vi "Admin (2).vi"() -> ()   [LabVIEW 2020]
panel:
  out "Ban":i32
  out "Tab Control":enum32{"Login", "Admin"}(tab)
  in  "Ingresar":bool
  in  "Contraseña":string
  in  "Usuario":string
  in  "Terminar":bool
  in  "AddContraseña":string
  in  "addUsuario":string
  in  "Agregar":bool
  out "Sesion Iniciada Por:":string
  in  "Volver":bool
  in  "Lista":bool
  out "String":string
  in  "Eliminar":bool
  in  "Ingrese el usuario que desea eliminar":string
  in  "Borrar":bool
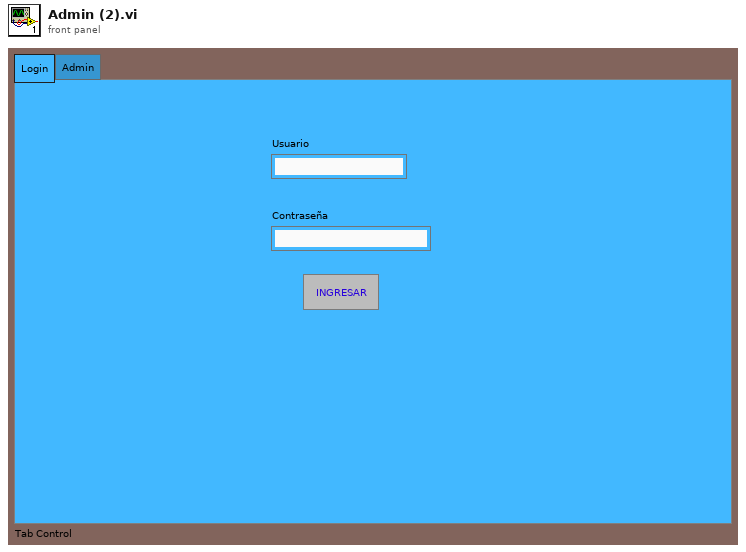
[diagram p1: front panel]
types:
  T1 = enum16{"open", "replace", "create", "open or create", "replace or create", "replace or create with confirmation"}
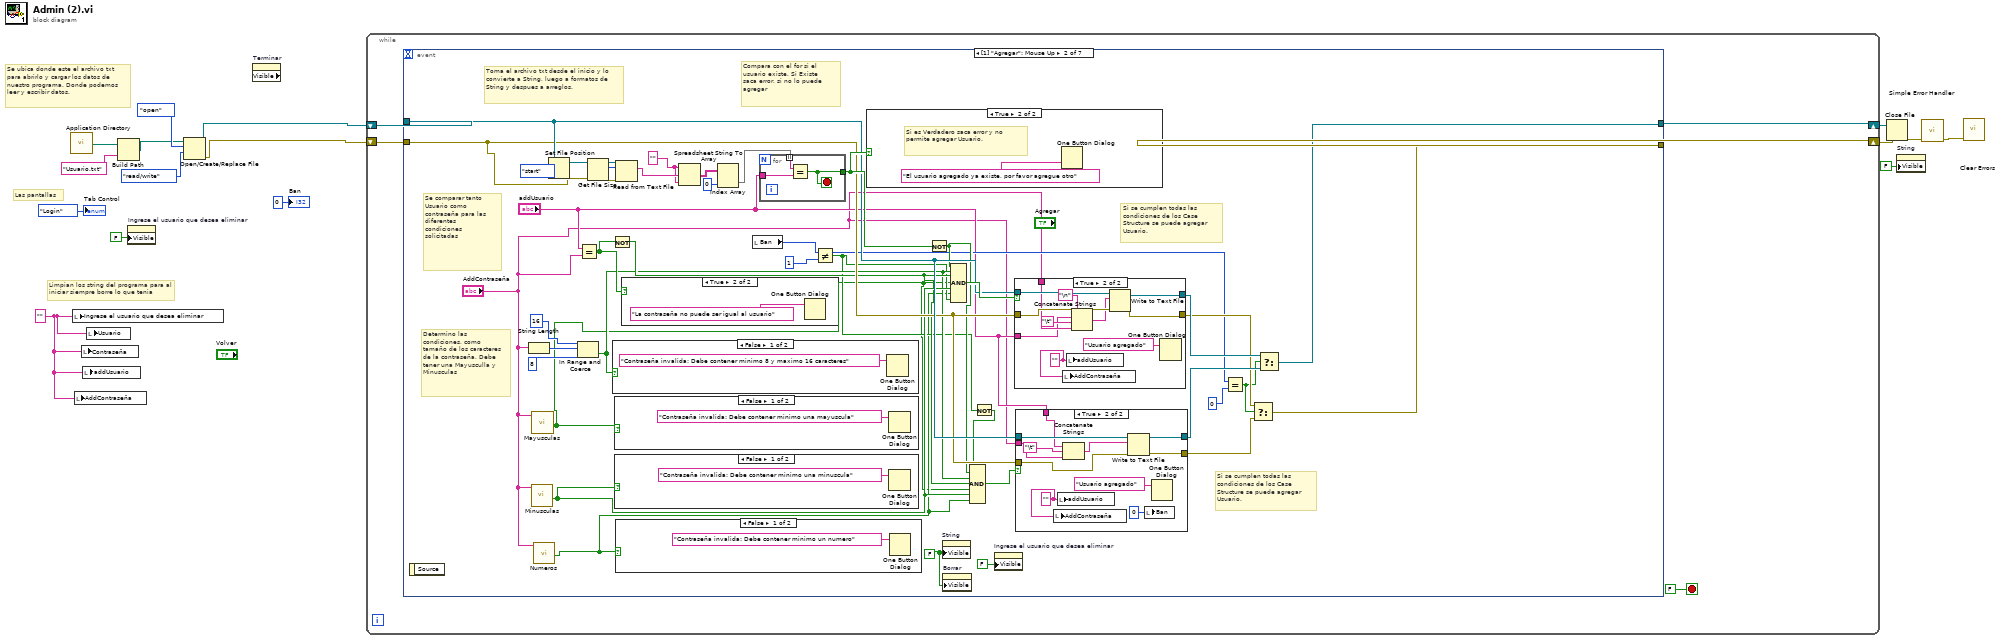
[diagram p0: block diagram]
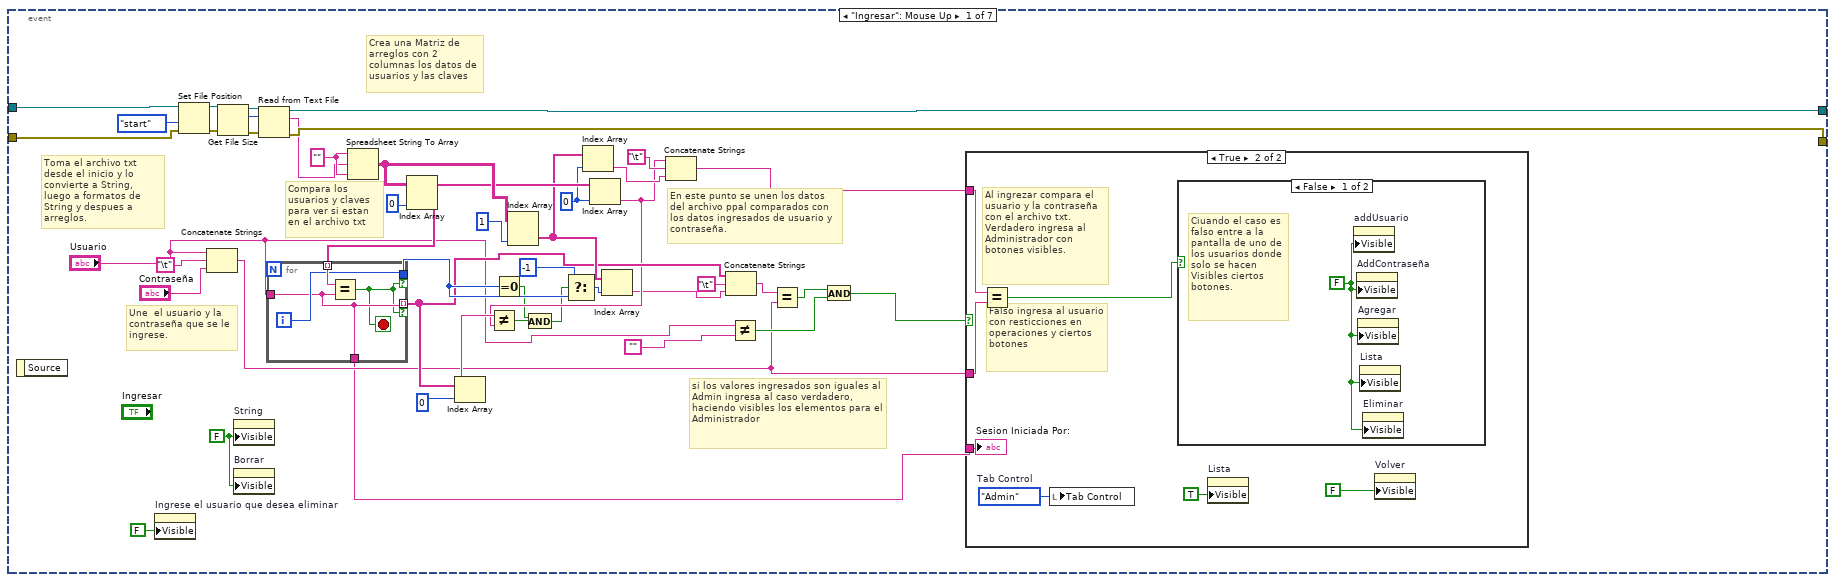
[diagram p2: hidden frame]
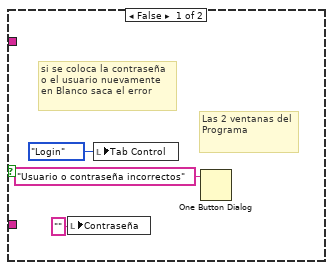
[diagram p3: hidden frame]
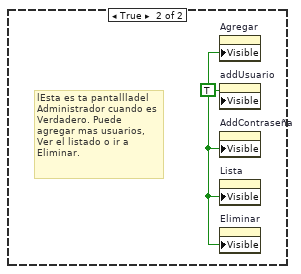
[diagram p4: hidden frame]
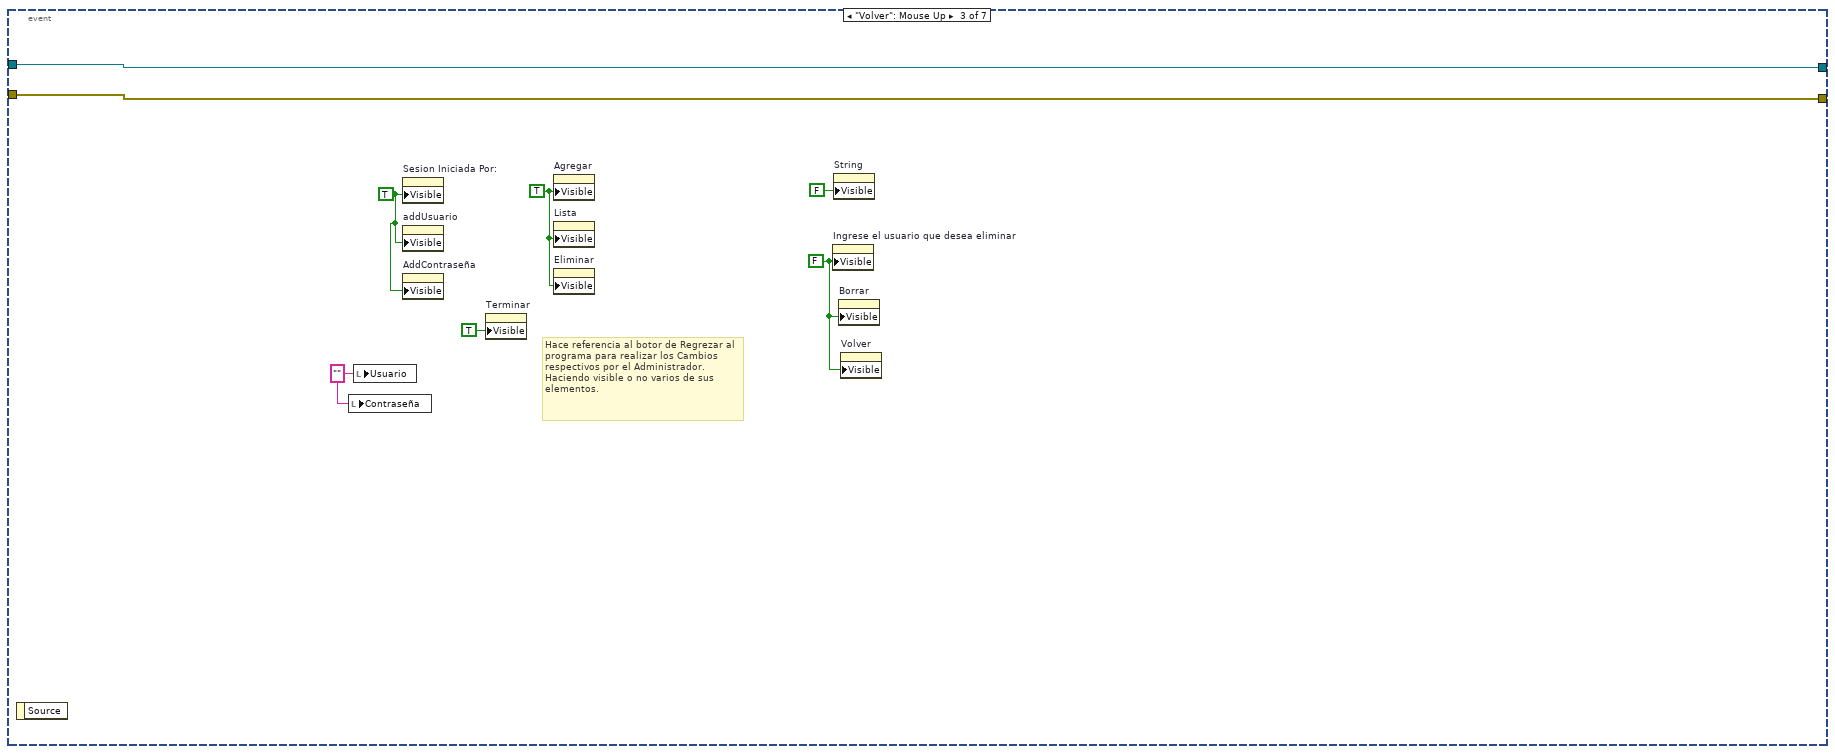
[diagram p13: hidden frame]
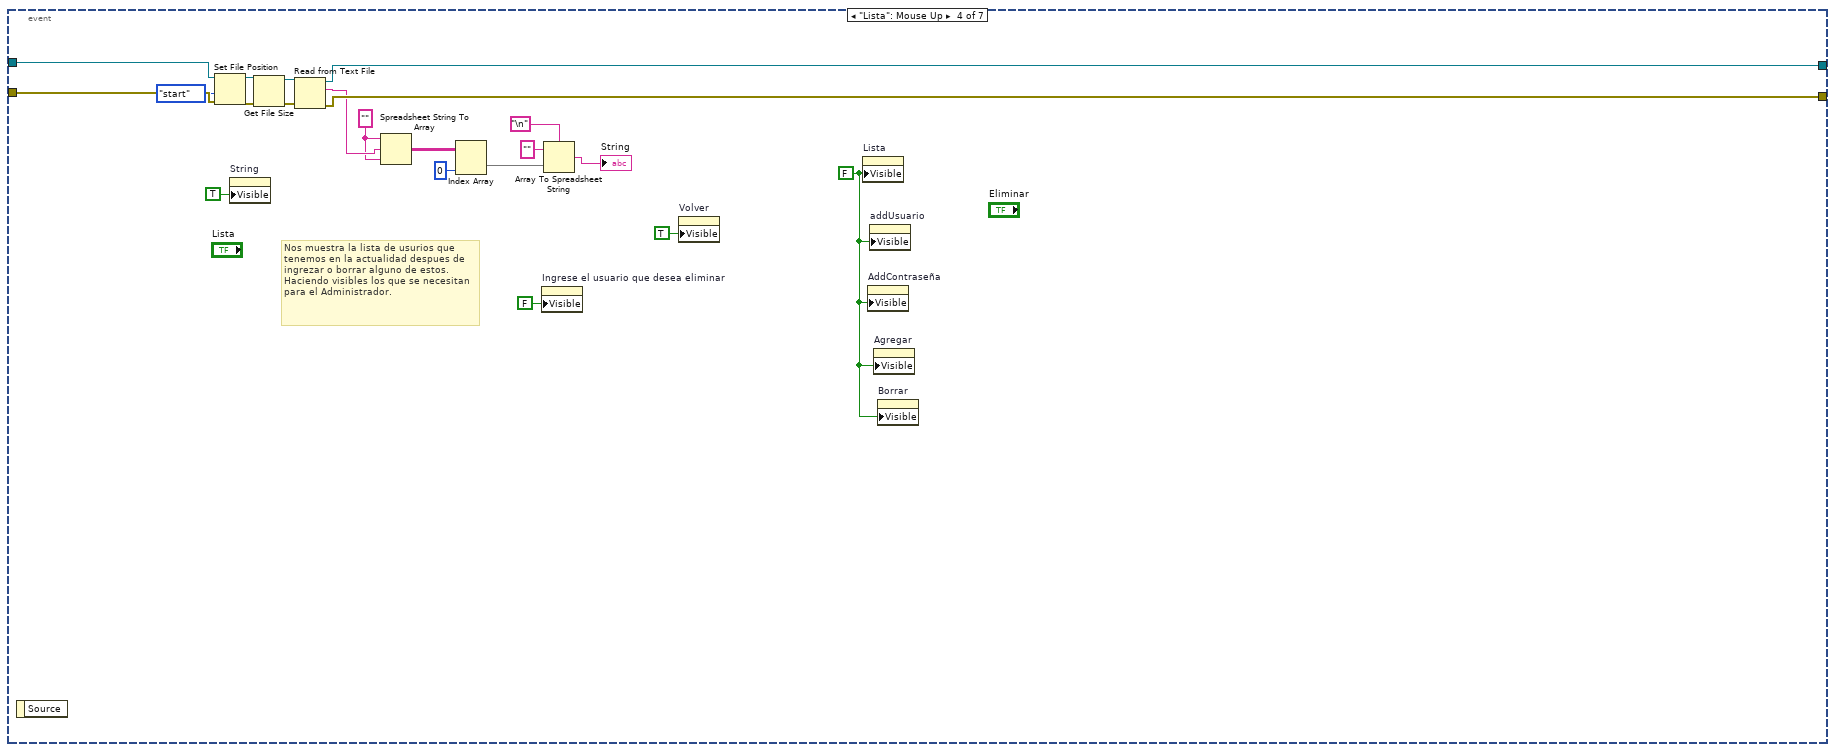
[diagram p14: hidden frame]
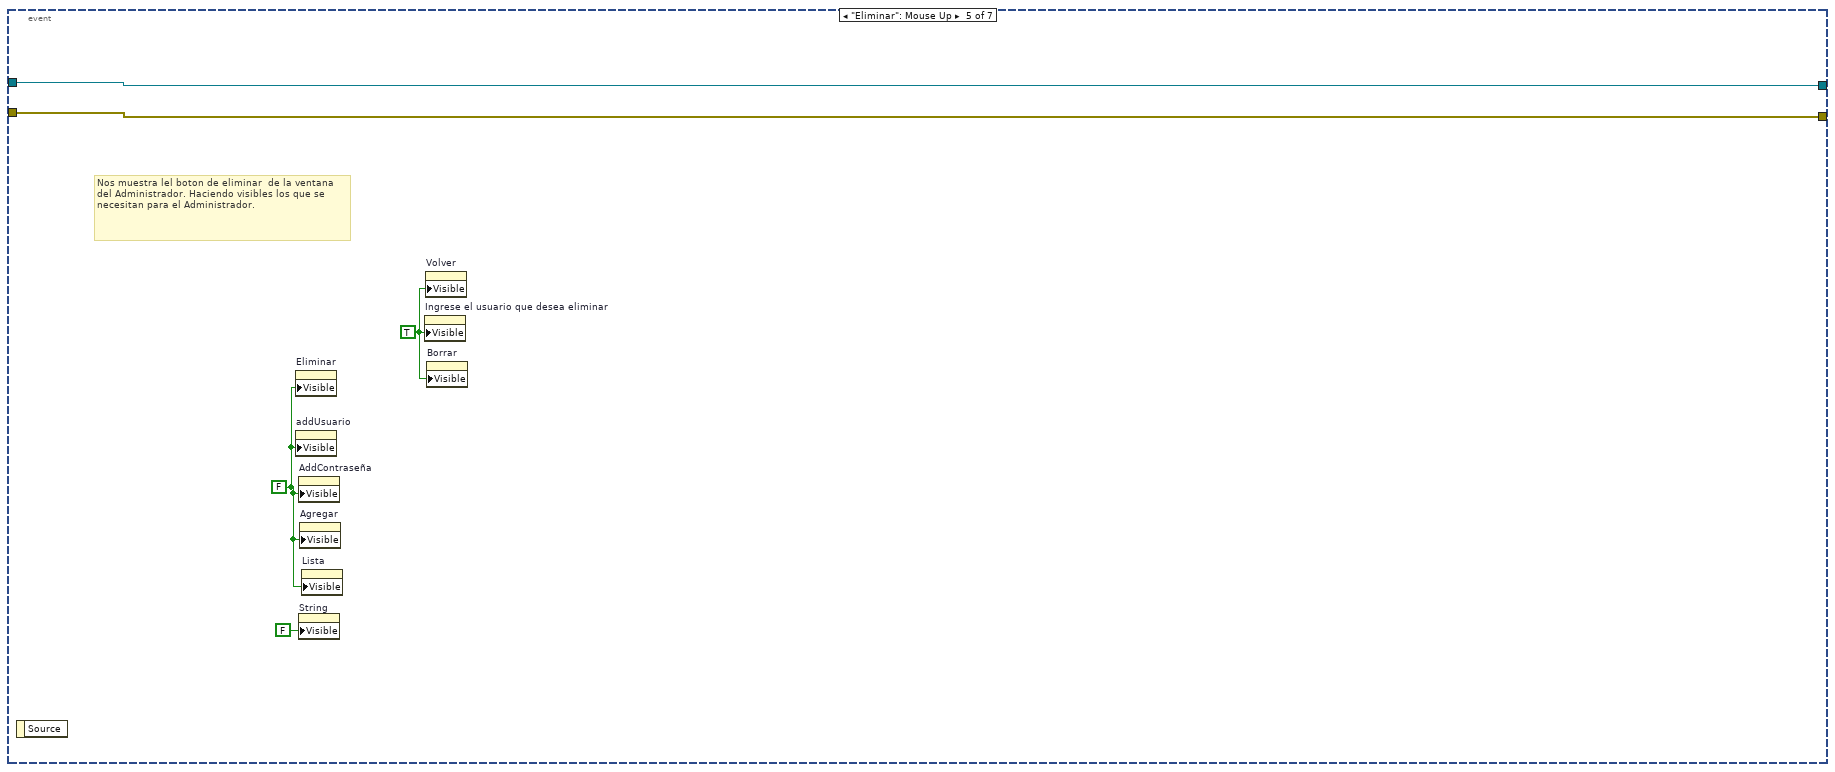
[diagram p15: hidden frame]
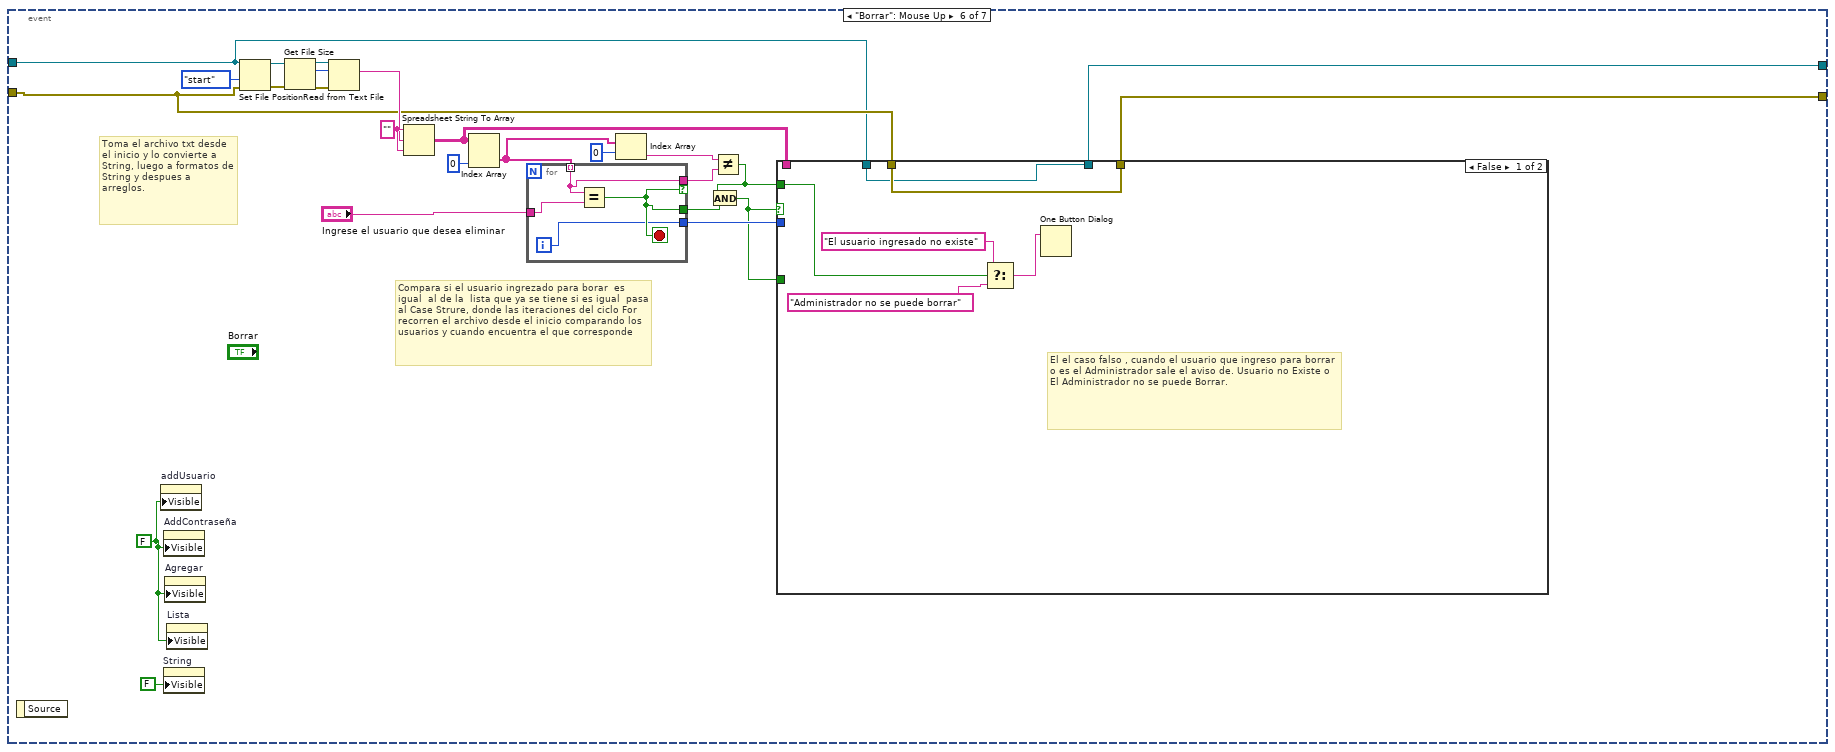
[diagram p16: hidden frame]
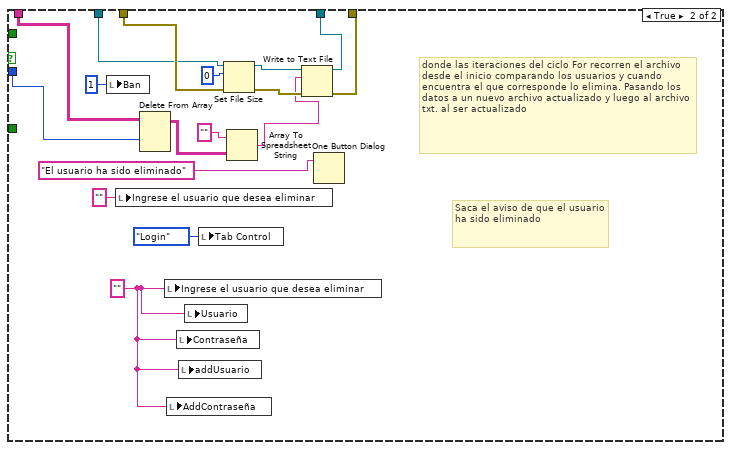
[diagram p17: hidden frame]
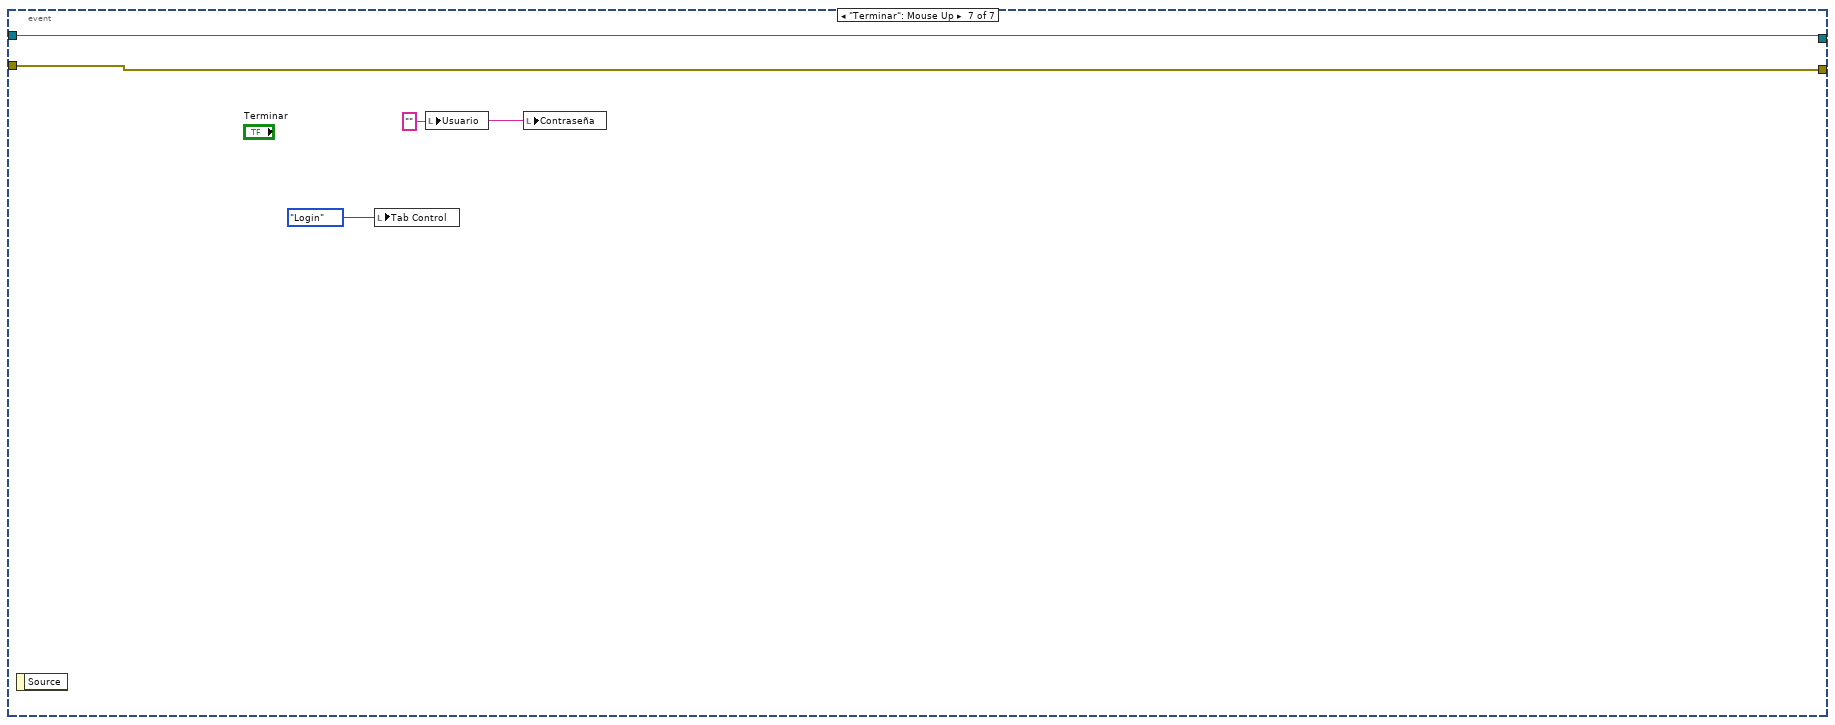
[diagram p18: hidden frame]
diagram:
  w6 = "" ("Usuario")
  # "Las pantallas"
  # "Limpian los string del programa para al iniciar siempre borre lo que tenia"
  # "Se ubica donde este el archivo txt para abrirlo y cargar los datos de nuestro programa. Donde podemos leer y escribir datos."
  n1 = call <vilib>:"Application Directory.vi"() -> ("Application Directory"=w16:path)
  n2 = local write "Ingrese el usuario que desea eliminar"(w6) -> ()
  n3 = local write "AddContraseña"(w6) -> ()
  n4 = local write "Contraseña"(w6) -> ()
  n5 = local write "addUsuario"(w6) -> ()
  n6 = local write "Usuario"(w6) -> ()
  n7 = Build Path(base path=w16, name or relative path="Usuario.txt") -> (appended path=w1:path)
  n8 = property on="Ingrese el usuario que desea eliminar" class="Str"("Visible"=FALSE) -> ()  [unwired: 2 in, 2 out]
  n9 = Open/Create/Replace File(file path (use dialog)=w1, operation (0:open)=T1."open", access (0:read/write)=enum16{"read/write", "read-only", "write-only"}."read/write") -> (refnum out=w4:refnum<file>, error out=w5:errorcluster)  [unwired: 3 in, 1 out]
  n10 = property on="Terminar" class="Bool (strict)" props=["Visible"]() -> ()  [unwired: 2 in, 3 out]
  n11 = while {
    shift-right: [w18] -> w10
    shift-left: w4 -> [w20]
    shift-right: [w17] -> w9
    shift-left: w5 -> [w19]
    stop <- FALSE stop-if-true
    n12 = event shown="[1] \"Agregar\": Mouse Up" {
      selector: _ -> [_ _ _ _ _ _ _]
      dyn-events: _ -> [_ _ _ _ _ _ _]
      timeout: _ -> [_ _ _ _ _ _ _]
      tunnel: w20 -> [w66 w104 w166 w186 w193 w203 w248]
      tunnel: w19 -> [w64 w103 w165 w183 w192 w204 w247]
      tunnel: [w42 w93 w166 w168 w193 w201 w248] -> w18
      tunnel: [w58 w90 w165 w181 w192 w202 w247] -> w17
      event "Ingresar": Mouse Up {
        w43 = FALSE ("Visible")
        w49 = 0 ("index")
        w56 = "" ("format string")
        # "En este punto se unen los datos del archivo ppal comparados con  los datos ingresados de usuario y contraseña."
        # "si los valores ingresados son iguales al  Admin ingresa al caso verdadero, haciendo visibles los elementos para el Administrador"
        # "Compara los usuarios y claves para ver si estan en el archivo txt"
        # "Une  el usuario y la contraseña que se le ingrese."
        # "Crea una Matriz de arreglos con 2 columnas los datos de usuarios y las claves"
        # "Toma el archivo txt desde el inicio y lo convierte a String, luego a formatos de String y despues a arreglos."
        n13 = event-data() -> ()  [unwired: 1 in, 1 out]
        n14 = property on="Ingrese el usuario que desea eliminar" class="Str"("Visible"=FALSE) -> ()  [unwired: 2 in, 2 out]
        n15 = Set File Position(refnum=w66, from (0:start)=enum16{"start", "end", "current"}."start", error in=w64) -> (refnum out=w62:refnum<file>, error out=w63:errorcluster)  [unwired: 1 in]
        n16 = Concatenate Strings "Concatenate Strings"("Usuario", "\t", "Contraseña") -> (w28:string)
        n17 = Get File Size(file=w62, error in=w63) -> (refnum out=w61:refnum<file>, size (in bytes)=w60:i64, 0:w59:errorcluster)
        n18 = property on="String" class="Str"("Visible"=w43) -> ()  [unwired: 2 in, 2 out]
        n19 = property on="Borrar" class="Bool (strict)"("Visible"=w43) -> ()  [unwired: 2 in, 2 out]
        n20 = Read from Text File(file (use dialog)=w61, count=w60, error in=w59) -> (refnum out=w42:refnum<file>, text=w53:string, error out=w58:errorcluster)  [unwired: 1 in, 1 out]
        n21 = Spreadsheet String To Array(format string=w56, spreadsheet string=w53, array type (2D Dbl)=w56) -> (array=w51:string[][])  [unwired: 1 in]
        n22 = Index Array "Index Array"(array=w51, index (col)=0 ("disabled index (col)")) -> (element=w50:string[])  [unwired: 1 in]
        n23 = for {
          tunnel: w50 -> [w70] mode=indexing
          tunnel: "Usuario" -> [w68]
          tunnel: [w68] -> w38 mode=indexing if=w67
          tunnel: [w69] -> w40 if=w67
          tunnel: [w68] -> w22
          i -> [w69]
          stop <- w67 stop-if-true
          n24 = Equal?(x=w70, y=w68) -> (x = y?=w67:bool)
        }
        n25 = Index Array "Index Array"(array=w38, index=0) -> (element=w36:string)
        n26 = Equal To 0?(x=w40) -> (x = 0?=w33:bool)
        n27 = Index Array "Index Array"(array=w51, index (col)=1 ("disabled index (col)")) -> (element=w45:string[])  [unwired: 1 in]
        n28 = Index Array "Index Array"(array=w45, index=w49) -> (element=w48:string)
        n29 = Index Array(array=w50, index=w49) -> (element=w35:string)
        n30 = Not Equal?(x=w36, y=w35) -> (x != y?=w34:bool)
        n31 = And(x=w33, y=w34) -> (x .and. y?=w32:bool)
        n32 = Select(t=-1, s=w32, f=w40) -> (s? t:f=w39:i32)
        n33 = Index Array(array=w45, index=w39) -> (element=w25:string)
        n34 = Concatenate Strings(w35, "\t", w48) -> (w46:string)
        n35 = Concatenate Strings "Concatenate Strings"(w38, "\t", w25) -> (w29:string)
        n36 = Not Equal?(x="Usuario", y="") -> (x != y?=w31:bool)
        n37 = Equal?(x=w29, y=w28) -> (x = y?=w26:bool)
        n38 = And(x=w26, y=w31) -> (x .and. y?=w30:bool)
        n39 = case shown="True" w30 {
          tunnel: w28 -> [_ w80]
          tunnel: w46 -> [_ w79]
          tunnel: w22 -> [_ w78]
          frame False {
            # "Las 2 ventanas del   Programa"
            # "si se coloca la contraseña o el usuario nuevamente en Blanco saca el error"
            n40 = local write "Contraseña"("" ("Usuario")) -> ()
            n41 = local write "Tab Control"(enum32{"Login", "Admin"}."Login" ("Tab Control")) -> ()
            n42 = One Button Dialog(message="Usuario o contraseña incorrectos") -> ()  [unwired: 1 in, 1 out]
          }
          frame True {
            w75 = enum32{"Login", "Admin"}."Admin"  # Tab Control
            # "Falso ingresa al usuario con resticciones en operaciones y ciertos botones"
            # "Al ingrezar compara el usuario y la contraseña con el archivo txt.  Verdadero ingresa al Administrador con botones visibles."
            n43 = Equal?(x=w79, y=w80) -> (x = y?=w76:bool)
            n44 = local write "Tab Control"(w75) -> ()
            n45 = case shown="False" w76 {
              frame False {
                w81 = FALSE ("Visible")
                # "Ciuando el caso es falso entre a la pantalla de uno de los usuarios donde  solo se hacen Visibles ciertos botones."
                n46 = property on="addUsuario" class="Str"("Visible"=w81) -> ()  [unwired: 2 in, 2 out]
                n47 = property on="AddContraseña" class="Str"("Visible"=w81) -> ()  [unwired: 2 in, 2 out]
                n48 = property on="Agregar" class="Bool (strict)"("Visible"=w81) -> ()  [unwired: 2 in, 2 out]
                n49 = property on="Lista" class="Bool (strict)"("Visible"=w81) -> ()  [unwired: 2 in, 2 out]
                n50 = property on="Eliminar" class="Bool (strict)"("Visible"=w81) -> ()  [unwired: 2 in, 2 out]
              }
              frame True {
                w82 = TRUE ("Visible")
                # "lEsta es ta pantallladel Administrador cuando es Verdadero. Puede agregar mas usuarios, Ver el listado o ir a Eliminar."
                n51 = property on="Agregar" class="Bool (strict)"("Visible"=w82) -> ()  [unwired: 2 in, 2 out]
                n52 = property on="addUsuario" class="Str"("Visible"=w82) -> ()  [unwired: 2 in, 2 out]
                n53 = property on="AddContraseña" class="Str"("Visible"=w82) -> ()  [unwired: 2 in, 2 out]
                n54 = property on="Lista" class="Bool (strict)"("Visible"=w82) -> ()  [unwired: 2 in, 2 out]
                n55 = property on="Eliminar" class="Bool (strict)"("Visible"=w82) -> ()  [unwired: 2 in, 2 out]
              }
            }
            n56 = property on="Lista" class="Bool (strict)"("Visible"=TRUE) -> ()  [unwired: 2 in, 2 out]
            n57 = property on="Volver" class="Bool (strict)"("Visible"=FALSE) -> ()  [unwired: 2 in, 2 out]
            "Sesion Iniciada Por:" <- w78
          }
        }
      }
      event "Agregar": Mouse Up {
        w106 = FALSE ("Visible")
        w112 = "" ("format string")
        # "Si se cumplen todas las condiciones de los Case Structure se puede agregar Usuario."
        # "Si se cumplen todas las condiciones de los Case Structure se puede agregar Usuario."
        # "Determino las condiciones, como tamaño de los caracteres de la contraseña, Debe tener una Mayusculla y Minusculas"
        # "Se comparar tanto Usuario como contraseña para las diferentes condiciones solicitadas"
        # "Compara con el for si el usuario existe. Si Existe saca error, si no lo puede agregar"
        # "Toma el archivo txt desde el inicio y lo convierte a String, luego a formatos de String y despues a arreglos."
        n58 = event-data() -> ()  [unwired: 1 in, 1 out]
        n59 = String Length(string="AddContraseña") -> (length=w122:i32)
        n60 = call "Minusculas.vi"("Palabra"="AddContraseña") -> ("Boolean"=w102:bool)  [unwired: 8 in, 2 out]
        n61 = call "Mayusculas.vi"("Palabra"="AddContraseña") -> ("Boolean"=w83:bool)  [unwired: 8 in, 2 out]
        n62 = call "Numeros.vi"("Palabra"="AddContraseña") -> ("Boolean"=w84:bool)  [unwired: 8 in, 2 out]
        n63 = Set File Position(refnum=w104, from (0:start)=enum16{"start", "end", "current"}."start", error in=w103) -> (refnum out=w115:refnum<file>, error out=w118:errorcluster)  [unwired: 1 in]
        n64 = In Range and Coerce(upper limit=16, x=w122, lower limit=8) -> (In Range?=w100:bool)  [unwired: 1 out]
        n65 = Equal?(x="addUsuario", y="AddContraseña") -> (x = y?=w121:bool)
        n66 = Get File Size(file=w115, error in=w118) -> (refnum out=w116:refnum<file>, size (in bytes)=w119:i64, 0:w117:errorcluster)
        n67 = Not(x=w121) -> (.not. x?=w101:bool)
        n68 = case shown="False" w100 {
          frame False {
            n69 = One Button Dialog(message="Contraseña invalida: Debe contener minimo 8 y maximo 16 caracteres") -> ()  [unwired: 1 in, 1 out]
          }
          frame True {
          }
        }
        n70 = case shown="False" w83 {
          frame False {
            n71 = One Button Dialog(message="Contraseña invalida: Debe contener minimo una mayuscula") -> ()  [unwired: 1 in, 1 out]
          }
          frame True {
          }
        }
        n72 = case shown="False" w102 {
          frame False {
            n73 = One Button Dialog(message="Contraseña invalida: Debe contener minimo una minuscula") -> ()  [unwired: 1 in, 1 out]
          }
          frame True {
          }
        }
        n74 = Read from Text File(file (use dialog)=w116, count=w119, error in=w117) -> (text=w113:string)  [unwired: 1 in, 3 out]
        n75 = case shown="False" w84 {
          frame False {
            n76 = One Button Dialog(message="Contraseña invalida: Debe contener minimo un numero") -> ()  [unwired: 1 in, 1 out]
          }
          frame True {
          }
        }
        n77 = case shown="True" w121 {
          frame False {
            # "Si no son iguales se pueden agregar al  Programa"
          }
          frame True {
            n78 = One Button Dialog(message="La contraseña no puede ser igual al usuario") -> ()  [unwired: 1 in, 1 out]
          }
        }
        n79 = Spreadsheet String To Array(format string=w112, spreadsheet string=w113, array type (2D Dbl)=w112) -> (array=w111:string[][])  [unwired: 1 in]
        n80 = Index Array(array=w111, index (col)=0 ("disabled index (col)")) -> (element=w109:string[])  [unwired: 1 in]
        n81 = local read "Ban"() -> (w87:i32)
        n82 = for {
          tunnel: "addUsuario" -> [w141]
          tunnel: w109 -> [w140] mode=indexing
          tunnel: [w139] -> w108
          stop <- w139 stop-if-true
          n83 = Equal?(x=w140, y=w141) -> (x = y?=w139:bool)
        }
        n84 = Not Equal?(x=w87, y=1) -> (x != y?=w98:bool)
        n85 = case shown="True" w108 {
          frame False {
            # "Si es Falso lo Puede Agregar ur¿suario en la base de Datos"
          }
          frame True {
            # "Si es Verdadero saca error y no permite agregar Usuario."
            n86 = One Button Dialog(message="El usuario agregado ya existe, por favor agregue otro") -> ()  [unwired: 1 in, 1 out]
          }
        }
        n87 = Not(x=w108) -> (.not. x?=w99:bool)
        n88 = property on="String" class="Str"("Visible"=w106) -> ()  [unwired: 2 in, 2 out]
        n89 = property on="Borrar" class="Bool (strict)"("Visible"=w106) -> ()  [unwired: 2 in, 2 out]
        n90 = Compound Arithmetic op=AND(w99, w100, w101, w83, w102, w84, w98) -> (w120:bool)
        n91 = Not(x=w98) -> (.not. x?=w97:bool)
        n92 = Compound Arithmetic op=AND(w97, w99, w100, w101, w83, w102, w84) -> (w96:bool)
        n93 = property on="Ingrese el usuario que desea eliminar" class="Str"("Visible"=FALSE) -> ()  [unwired: 2 in, 2 out]
        n94 = case shown="True" w120 {
          tunnel: w104 -> [w146 w157]
          tunnel: w103 -> [w145 w156]
          tunnel: [w146 w155] -> w95
          tunnel: [w145 w154] -> w92
          tunnel: "addUsuario" -> [_ w147]
          tunnel: "AddContraseña" -> [_ w153]
          frame False {
          }
          frame True {
            w148 = "" ("addUsuario")
            n95 = local write "AddContraseña"(w148) -> ()
            n96 = local write "addUsuario"(w148) -> ()
            n97 = Concatenate Strings("\n", w147, "\t", w153) -> (w152:string)
            n98 = Write to Text File(file (use dialog)=w157, text=w152, error in=w156) -> (refnum out=w155:refnum<file>, error out=w154:errorcluster)  [unwired: 1 in, 1 out]
            n99 = One Button Dialog(message="Usuario agregado") -> ()  [unwired: 1 in, 1 out]
          }
        }
        n100 = case shown="True" w96 {
          tunnel: w104 -> [w126 w133]
          tunnel: w103 -> [w125 w132]
          tunnel: [w126 w131] -> w94
          tunnel: [w125 w130] -> w91
          tunnel: "addUsuario" -> [_ w128]
          tunnel: "AddContraseña" -> [_ w127]
          frame False {
          }
          frame True {
            w137 = "" ("addUsuario")
            n101 = local write "AddContraseña"(w137) -> ()
            n102 = local write "addUsuario"(w137) -> ()
            n103 = Concatenate Strings(w128, "\t", w127) -> (w135:string)
            n104 = Write to Text File(file (use dialog)=w133, text=w135, error in=w132) -> (refnum out=w131:refnum<file>, error out=w130:errorcluster)  [unwired: 1 in, 1 out]
            n105 = local write "Ban"(0 ("Ban")) -> ()
            n106 = One Button Dialog(message="Usuario agregado") -> ()  [unwired: 1 in, 1 out]
          }
        }
        n107 = Equal?(x=w87, y=0) -> (x = y?=w88:bool)
        n108 = Select(t=w92, s=w88, f=w91) -> (s? t:f=w90:errorcluster)
        n109 = Select(t=w95, s=w88, f=w94) -> (s? t:f=w93:refnum<file>)
      }
      event "Volver": Mouse Up {
        w162 = TRUE ("Visible")
        w163 = TRUE ("Visible")
        w160 = FALSE ("Visible")
        w167 = "" ("Usuario")
        # "Hace referencia al botor de Regrezar al programa para realizar los Cambios respectivos por el Administrador.  Haciendo visible o no varios de sus elementos."
        n110 = event-data() -> ()  [unwired: 1 in, 1 out]
        n111 = local write "Contraseña"(w167) -> ()
        n112 = local write "Usuario"(w167) -> ()
        n113 = property on="Sesion Iniciada Por:" class="Str"("Visible"=w163) -> ()  [unwired: 2 in, 2 out]
        n114 = property on="addUsuario" class="Str"("Visible"=w163) -> ()  [unwired: 2 in, 2 out]
        n115 = property on="AddContraseña" class="Str"("Visible"=w163) -> ()  [unwired: 2 in, 2 out]
        n116 = property on="Terminar" class="Bool (strict)"("Visible"=TRUE) -> ()  [unwired: 2 in, 2 out]
        n117 = property on="Agregar" class="Bool (strict)"("Visible"=w162) -> ()  [unwired: 2 in, 2 out]
        n118 = property on="Lista" class="Bool (strict)"("Visible"=w162) -> ()  [unwired: 2 in, 2 out]
        n119 = property on="Eliminar" class="Bool (strict)"("Visible"=w162) -> ()  [unwired: 2 in, 2 out]
        n120 = property on="Ingrese el usuario que desea eliminar" class="Str"("Visible"=w160) -> ()  [unwired: 2 in, 2 out]
        n121 = property on="String" class="Str"("Visible"=FALSE) -> ()  [unwired: 2 in, 2 out]
        n122 = property on="Borrar" class="Bool (strict)"("Visible"=w160) -> ()  [unwired: 2 in, 2 out]
        n123 = property on="Volver" class="Bool (strict)"("Visible"=w160) -> ()  [unwired: 2 in, 2 out]
      }
      event "Lista": Mouse Up {
        w170 = FALSE ("Visible")
        w179 = "" ("format string")
        # "Nos muestra la lista de usurios que tenemos en la actualidad despues de ingrezar o borrar alguno de estos. Haciendo visibles los que se necesitan para el Administrador."
        n124 = event-data() -> ()  [unwired: 1 in, 1 out]
        n125 = Set File Position(refnum=w186, from (0:start)=enum16{"start", "end", "current"}."start", error in=w183) -> (refnum out=w188:refnum<file>, error out=w184:errorcluster)  [unwired: 1 in]
        n126 = property on="String" class="Str"("Visible"=TRUE) -> ()  [unwired: 2 in, 2 out]
        n127 = Get File Size(file=w188, error in=w184) -> (refnum out=w187:refnum<file>, 0:w185:errorcluster)  [unwired: 1 out]
        n128 = Read from Text File(file (use dialog)=w187, error in=w185) -> (refnum out=w168:refnum<file>, text=w180:string, error out=w181:errorcluster)  [unwired: 2 in, 1 out]
        n129 = Spreadsheet String To Array(format string=w179, spreadsheet string=w180, array type (2D Dbl)=w179) -> (array=w178:string[][])  [unwired: 1 in]
        n130 = Index Array(array=w178, index (col)=0 ("disabled index (col)")) -> (element=w175:string[])  [unwired: 1 in]
        n131 = property on="Ingrese el usuario que desea eliminar" class="Str"("Visible"=FALSE) -> ()  [unwired: 2 in, 2 out]
        n132 = Array To Spreadsheet String(delimiter (Tab)="\n", array=w175, 3:"" ("format string")) -> (spreadsheet string=→"String":string)
        n133 = property on="Volver" class="Bool (strict)"("Visible"=TRUE) -> ()  [unwired: 2 in, 2 out]
        n134 = property on="Lista" class="Bool (strict)"("Visible"=w170) -> ()  [unwired: 2 in, 2 out]
        n135 = property on="AddContraseña" class="Str"("Visible"=w170) -> ()  [unwired: 2 in, 2 out]
        n136 = property on="addUsuario" class="Str"("Visible"=w170) -> ()  [unwired: 2 in, 2 out]
        n137 = property on="Agregar" class="Bool (strict)"("Visible"=w170) -> ()  [unwired: 2 in, 2 out]
        n138 = property on="Borrar" class="Bool (strict)"("Visible"=w170) -> ()  [unwired: 2 in, 2 out]
      }
      event "Eliminar": Mouse Up {
        w190 = FALSE ("Visible")
        w189 = TRUE ("Visible")
        # "Nos muestra lel boton de eliminar  de la ventana del Administrador. Haciendo visibles los que se necesitan para el Administrador."
        n139 = event-data() -> ()  [unwired: 1 in, 1 out]
        n140 = property on="Eliminar" class="Bool (strict)"("Visible"=w190) -> ()  [unwired: 2 in, 2 out]
        n141 = property on="addUsuario" class="Str"("Visible"=w190) -> ()  [unwired: 2 in, 2 out]
        n142 = property on="AddContraseña" class="Str"("Visible"=w190) -> ()  [unwired: 2 in, 2 out]
        n143 = property on="String" class="Str"("Visible"=FALSE) -> ()  [unwired: 2 in, 2 out]
        n144 = property on="Agregar" class="Bool (strict)"("Visible"=w190) -> ()  [unwired: 2 in, 2 out]
        n145 = property on="Lista" class="Bool (strict)"("Visible"=w190) -> ()  [unwired: 2 in, 2 out]
        n146 = property on="Ingrese el usuario que desea eliminar" class="Str"("Visible"=w189) -> ()  [unwired: 2 in, 2 out]
        n147 = property on="Volver" class="Bool (strict)"("Visible"=w189) -> ()  [unwired: 2 in, 2 out]
        n148 = property on="Borrar" class="Bool (strict)"("Visible"=w189) -> ()  [unwired: 2 in, 2 out]
      }
      event "Borrar": Mouse Up {
        w210 = "" ("format string")
        w218 = FALSE ("Visible")
        # "Compara si el usuario ingrezado para borar  es igual  al de la  lista que ya se tiene si es igual  pasa al Case Strure, donde las iteraciones del ciclo For recorren el archivo desde el inicio comparando los usuarios y cuando encuentra el que corresponde"
        # "Toma el archivo txt desde el inicio y lo convierte a String, luego a formatos de String y despues a arreglos."
        n149 = event-data() -> ()  [unwired: 1 in, 1 out]
        n150 = property on="addUsuario" class="Str"("Visible"=w218) -> ()  [unwired: 2 in, 2 out]
        n151 = property on="AddContraseña" class="Str"("Visible"=w218) -> ()  [unwired: 2 in, 2 out]
        n152 = property on="String" class="Str"("Visible"=FALSE) -> ()  [unwired: 2 in, 2 out]
        n153 = property on="Agregar" class="Bool (strict)"("Visible"=w218) -> ()  [unwired: 2 in, 2 out]
        n154 = property on="Lista" class="Bool (strict)"("Visible"=w218) -> ()  [unwired: 2 in, 2 out]
        n155 = Set File Position(refnum=w203, from (0:start)=enum16{"start", "end", "current"}."start", error in=w204) -> (refnum out=w215:refnum<file>, error out=w214:errorcluster)  [unwired: 1 in]
        n156 = Get File Size(file=w215, error in=w214) -> (refnum out=w213:refnum<file>, size (in bytes)=w211:i64, 0:w212:errorcluster)
        n157 = Read from Text File(file (use dialog)=w213, count=w211, error in=w212) -> (text=w209:string)  [unwired: 1 in, 3 out]
        n158 = Spreadsheet String To Array(format string=w210, spreadsheet string=w209, array type (2D Dbl)=w210) -> (array=w206:string[][])  [unwired: 1 in]
        n159 = Index Array(array=w206, index (col)=0 ("disabled index (col)")) -> (element=w196:string[])  [unwired: 1 in]
        n160 = for {
          tunnel: w196 -> [w244] mode=indexing
          tunnel: "Ingrese el usuario que desea eliminar" -> [w245]
          tunnel: [w243] -> w198
          tunnel: [w244] -> w195 if=w243
          tunnel: [w242] -> w205
          i -> [w242]
          stop <- w243 stop-if-true
          n161 = Equal?(x=w244, y=w245) -> (x = y?=w243:bool)
        }
        n162 = Index Array(array=w196, index=0) -> (element=w199:string)
        n163 = Not Equal?(x=w199, y=w195) -> (x != y?=w194:bool)
        n164 = And(x=w194, y=w198) -> (x .and. y?=w197:bool)
        n165 = case shown="False" w197 {
          tunnel: w206 -> [_ w241]
          tunnel: w205 -> [_ w240]
          tunnel: w204 -> [w224 w237]
          tunnel: w203 -> [w223 w236]
          tunnel: [w224 w239] -> w202
          tunnel: [w223 w238] -> w201
          tunnel: w197 -> [_ _]
          tunnel: w194 -> [w221 _]
          frame False {
            # "El el caso falso , cuando el usuario que ingreso para borrar o es el Administrador sale el aviso de. Usuario no Existe o El Administrador no se puede Borrar."
            n166 = Select(t="El usuario ingresado no existe" ("message"), s=w221, f="Administrador no se puede borrar" ("message")) -> (s? t:f=w219:string)
            n167 = One Button Dialog(message=w219) -> ()  [unwired: 1 in, 1 out]
          }
          frame True {
            w225 = "" ("Usuario")
            # "Saca el aviso de que el usuario ha sido eliminado"
            # "donde las iteraciones del ciclo For recorren el archivo desde el inicio comparando los usuarios y cuando encuentra el que corresponde lo elimina. Pasando los datos a un nuevo archivo actualizado y luego al archivo txt. al ser actualizado"
            n168 = local write "Ban"(1 ("Ban")) -> ()
            n169 = local write "Ingrese el usuario que desea eliminar"("" ("Ingrese el usuario que desea eliminar")) -> ()
            n170 = Delete From Array "Delete From Array"(array=w241, index (row)=w240) -> (array with subset deleted=w235:string[][])  [unwired: 2 in, 1 out]
            n171 = local write "Ingrese el usuario que desea eliminar"(w225) -> ()
            n172 = local write "AddContraseña"(w225) -> ()
            n173 = local write "Contraseña"(w225) -> ()
            n174 = local write "addUsuario"(w225) -> ()
            n175 = local write "Usuario"(w225) -> ()
            n176 = local write "Tab Control"(enum32{"Login", "Admin"}."Login" ("Tab Control")) -> ()
            n177 = Set File Size(4:w237, 6:i64 0 ("size (in bytes)"), 7:w236) -> (0:w232:errorcluster, 3:w233:refnum<file>)
            n178 = Array To Spreadsheet String(array=w235, 3:"") -> (spreadsheet string=w227:string)  [unwired: 1 in]
            n179 = Write to Text File(file (use dialog)=w233, text=w227, error in=w232) -> (refnum out=w238:refnum<file>, error out=w239:errorcluster)  [unwired: 1 in, 1 out]
            n180 = One Button Dialog(message="El usuario ha sido eliminado") -> ()  [unwired: 1 in, 1 out]
          }
        }
      }
      event "Terminar": Mouse Up {
        w246 = "" ("Usuario")
        n181 = event-data() -> ()  [unwired: 1 in, 1 out]
        n182 = local write "Tab Control"(enum32{"Login", "Admin"}."Login" ("Tab Control")) -> ()
        n183 = local write "Usuario"(w246) -> ()
        n184 = local write "Contraseña"(w246) -> ()
      }
    }
  }
  n185 = Close File(refnum=w10, error in=w9) -> (error out=w11:errorcluster)  [unwired: 1 out]
  n186 = property on="String" class="Str"("Visible"=FALSE) -> ()  [unwired: 2 in, 2 out]
  n187 = call <vilib>:"Simple Error Handler.vi"("error in (no error)"=w11) -> ("error out"=w12:errorcluster)  [unwired: 4 in, 4 out]
  n188 = call <vilib>:"Clear Errors.vi"("error in (no error)"=w12) -> ()  [unwired: 5 in, 2 out]
  "Tab Control" <- enum32{"Login", "Admin"}."Login" ("Tab Control")
  "Ban" <- 0 ("Ban")
